vi "Test_Complete_Core.vi"(8 "Vehicle":string, 9 "SMS Recipients":u32, 11 "File Name":string) -> ()   [LabVIEW 2014]
panel:
  out "Boolean array":bool[](array[boolean])
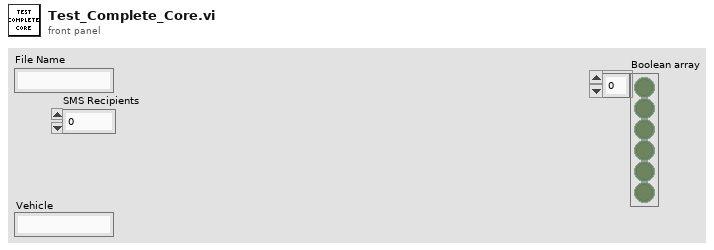
[diagram p1: front panel]
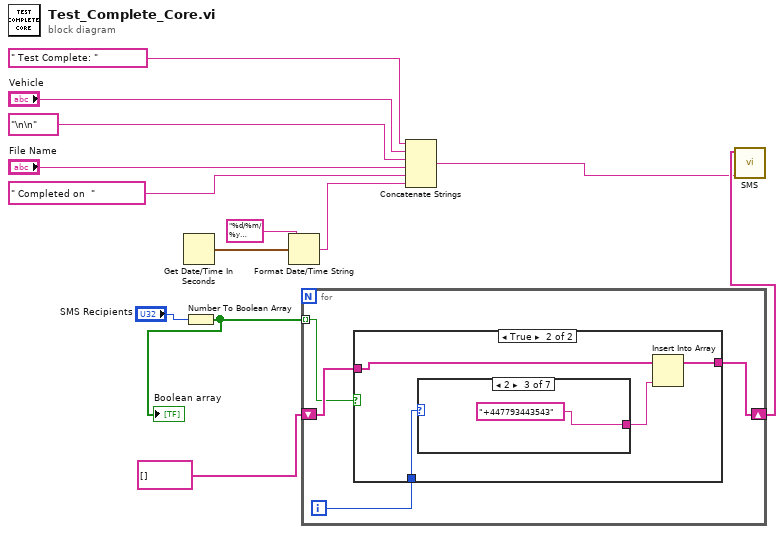
[diagram p0: block diagram]
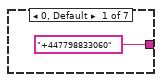
[diagram p3: hidden frame]
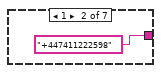
[diagram p4: hidden frame]
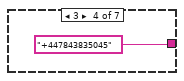
[diagram p5: hidden frame]
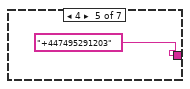
[diagram p6: hidden frame]
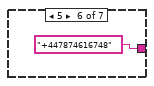
[diagram p7: hidden frame]
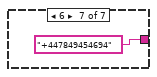
[diagram p8: hidden frame]
diagram:
  n1 = Get Date/Time In Seconds() -> (seconds since 1Jan1904=w13:timestamp)
  n2 = Number To Boolean Array(number="SMS Recipients") -> (Boolean array=w4:bool[])
  "Boolean array" <- w4
  n3 = Format Date/Time String(time format string (%c)="%d/%m/%y %H:%M:%S", seconds (now)=w13) -> (date/time string=w10:string)  [unwired: 1 in]
  n4 = for {
    tunnel: w4 -> [w16] mode=indexing
    shift-right: [w14] -> w2
    shift-left: string[] [] -> [w17]
    i -> [w15]
    n5 = case shown="True" w16 {
      tunnel: w17 -> [w18 w20]
      tunnel: w15 -> [_ w22]
      tunnel: [w18 w19] -> w14
      frame False {
      }
      frame True {
        n6 = case shown="2" w22 {
          tunnel: ["+447798833060" "+447411222598" "+447793443543" "+447843835045" "+447495291203" "+447874616748" "+447849454694"] -> w21
          frame 0, Default {
          }
          frame 1 {
          }
          frame 2 {
          }
          frame 3 {
          }
          frame 4 {
          }
          frame 5 {
          }
          frame 6 {
          }
        }
        n7 = Insert Into Array(array=w20, new element=w21) -> (w19:string[])  [unwired: 1 in]
      }
    }
  }
  n8 = Concatenate Strings(" Test Complete: " ("string"), "Vehicle", "\n\n" ("string"), "File Name", " Completed on  " ("string"), w10) -> (w1:string)
  n9 = call "SMS.vi"("text"=w1, "phoneNumbers"=w2) -> ()  [unwired: 10 in]
